vi "Can_Add.vi"(8 "error in (no error)":errorcluster, 11 "IB_Tree_Item_Proj_BuildSpecs in":refnum<class "IB_Tree_Item_Proj_BuildSpecs.lvclass">) -> (0 "error out":errorcluster, 2 "can add?":bool, 3 "IB_Tree_Item_Proj_BuildSpecs out":refnum<class "IB_Tree_Item_Proj_BuildSpecs.lvclass">)   [LabVIEW 2020, in "IB_Tree_Item_Proj_BuildSpecs.lvclass"]
uses:
  <vilib>/AppBuilder/IB_Classes/Tree_Item_Proj_BuildSpecs/IB_Tree_Item_Proj_BuildSpecs.lvclass
  <vilib>/AppBuilder/IB_Classes/Tree_Item_Proj_BuildSpecs/IB_Tree_Item_Proj_BuildSpecs.lvclass/IB_Tree_Item_Proj_BuildSpecs.ctl
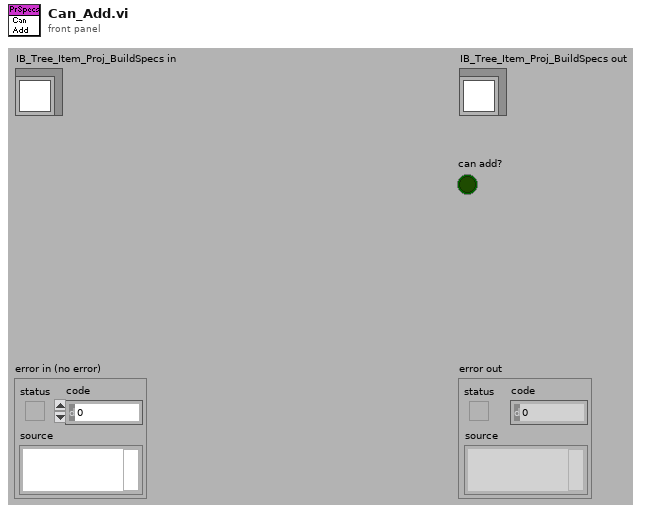
[diagram p1: front panel]
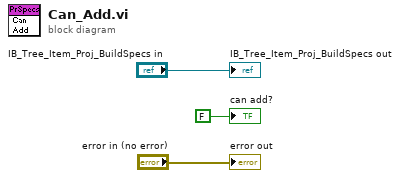
[diagram p0: block diagram]
diagram:
  "error out" <- "error in (no error)"
  "IB_Tree_Item_Proj_BuildSpecs out" <- "IB_Tree_Item_Proj_BuildSpecs in"
  "can add?" <- FALSE ("can add?")
